vi "Dashboard Main.vi"() -> ()   [LabVIEW 2011]
uses:
  gun/gun_motor_state.ctl
  gun/gun_tracking_mode.ctl
  dashboard_data_gun_fast.ctl
  gun/gun_rt_slow_upstream_data.ctl
  idg_trust_t.ctl
  dashboard_data_drivetrain.ctl
  drivetrain/gear_shift_state.ctl
  drivetrain/gear_internal_shift_state.ctl
  roller/roller_internal_state.ctl
  roller/roller_user_state.ctl
  joe_johnson/joe_johnson_state.ctl
  2012vision/Vision Instrumentation Control.ctl
  dashboard_return_data.ctl
  2012vision/Camera State.ctl
  dashboard_globals.vi
  <vilib>/vision/NI_Vision_Development_Module.lvlib
panel:
  in  "open_logger":bool
  out "Automode":string
  out "gun tracking mode":T1
  out "Shooter Control Mode":T2
  out "Gun Power":dbl
  out "Gun Speed":dbl
  out "Gun Speed Target":dbl
  in  "Debug Mode":enum16{"Show Targets", "Show Lines", "Show All"}(ring)
  in  "Threshold Range":cluster{"Lower value":sgl, "Upper value":sgl}={"Lower value"=217.0, "Upper value"=255.0} {"Upper value" format="%.2f"; "Lower value" format="%.2f"}
  out "error out":errorcluster
  out "Image":T3(plugin-control)
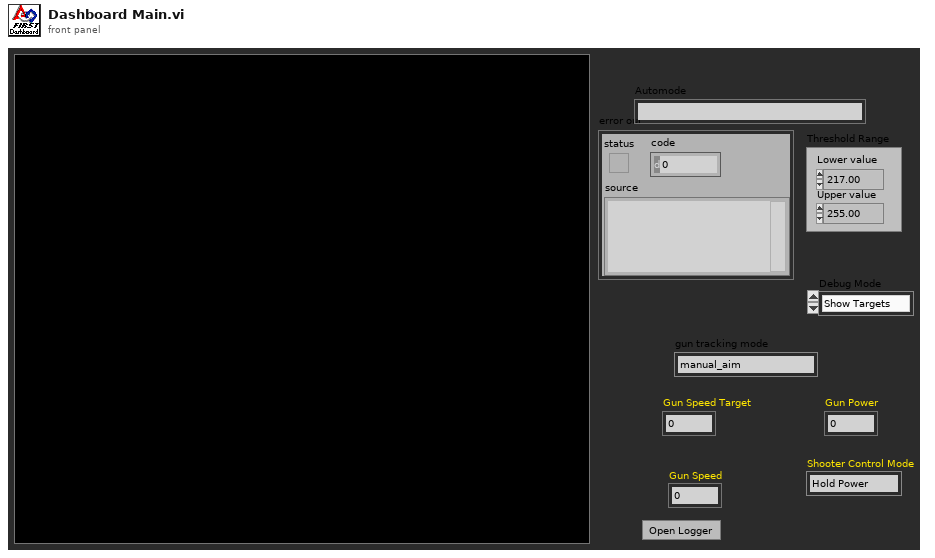
[diagram p1: front panel]
types:
  T1 = typedef "gun_tracking_mode.ctl" = enum16{"manual_aim", "auto_aim_camera", "preset_center_field", "preset_right_pocket", "preset_left_pocket", "align_center", "align_center_backwards", "auto_aim_key", "align_fold", "auton_custom", "preset_pass", "auto_aim_auton"}
  T2 = typedef "gun_motor_state.ctl" = enum16{"Hold Power", "Hold Speed", "Hold Distance", "Stop"}
  T3 = typedef "IMAQ Image.ctl" = refnum<image>
  T4 = typedef "dashboard_data_gun_fast.ctl" = cluster{"speed_setpoint":dbl, "speed_sensor":dbl, "gun_power":dbl, "gun_control_mode":T2, "gun_tracking_mode":T1}
  T5 = typedef "gun_rt_slow_upstream_data.ctl" = cluster{"turret":cluster{"turret_analog":dbl, "turret_angle":dbl, "turret_motor":dbl, "turret_idg_state":T6}, "hood":cluster{"hood_analog":dbl, "hood_angle":dbl, "hood_motor":dbl, "hood_idg_state":T6}}
  T6 = typedef "idg_trust_t.ctl" = enum16{"fault_move", "fault_high", "fault_low", "out_high", "out_low", "trust"}
  T7 = typedef "dashboard_data_drivetrain.ctl" = cluster{"left":cluster{"request":dbl, "enc_speed":dbl}, "right":cluster{"request":dbl, "enc_speed":dbl}, "gear shift state":T8, "gear shift internal state":T9}
  T8 = typedef "gear_shift_state.ctl" = enum16{"low", "high"}
  T9 = typedef "gear_internal_shift_state.ctl" = enum16{"low", "high", "low_peak", "high_peak"}
  T10 = typedef "roller_internal_state.ctl" = enum16{"idle", "bump", "full", "fire_intermediate", "fire_finish", "fire_entry", "fire_end", "fire_recover"}
  T11 = typedef "roller_user_state.ctl" = enum16{"off", "collect", "blow", "force suck"}
  T12 = typedef "joe_johnson_state.ctl" = enum16{"fold", "down", "up", "ramp", "bridge_lift", "manual", "ramp_stay"}
  T13 = cluster{"gun_fast":T4, "gun_slow":T5, "drivetrain_data":T7, "roller data":cluster{"roller internal state":T10, "roller user state":T11, "sws":cluster{"r_sw_b1":bool, "r_sw_b2":bool, "r_sw_b3":bool, "r_sw_gun":bool, "r_sw_low":bool}}, "joe_johnson_data":cluster{"analog":dbl, "input":dbl, "joe_johnson_state":T12, "idg_state":T6}}
  T14 = typedef "Image Type" = u32
  T15 = typedef "LVRectTypeDef.ctl" = cluster{"left":i16, "top":i16, "right":i16, "bottom":i16}
  T16 = cluster{"Competition mode":bool, "Robot Link":bool, "Autonomous":bool, "Enabled":bool, "E-Stop":bool}
  T17 = typedef "Vision Instrumentation Control.ctl" = cluster{"Draw Boxes":bool, "Draw Scores":bool, "Draw Lines":bool, "Draw Line Angles":bool, "Draw Targets":bool, "Draw Compound Crosshair":bool, "Draw Center Line":bool}
  T18 = enum32{"AutoM", "Close", "Dilate", "Erode", "Gradient", "Gradient in", "Gradient out", "HitMiss", "Open", "PClose", "POpen", "Thick", "Thin"}
  T19 = typedef "dashboard_return_data.ctl" = cluster{"Targetting Output":cluster{"X Position":dbl, "Distance":dbl, "Camera State":T20}, "Camera Error Status":errorcluster, "packet send timestamp":u32, "img process timestamp":u32}
  T20 = typedef "Camera State.ctl" = enum16{"No Targets", "Low Confidence", "Medium Confidence", "High Confidence", "Camera Error"}
  T21 = cluster{"Rect Coverage":dbl, "Aspect Ratio":dbl, "X Edge Strength":dbl, "Y Edge Strength":dbl}
  T22 = typedef "WPI_CameraImageSize.ctl" = enum16{"640x480", "320x240", "160x120"}
  T23 = cluster{"fps dashboard":i32, "compression dashboard":i32, "img size dashboard":T22}
  T24 = cluster{cluster{"Left":dbl, "Top":dbl, "Right":dbl, "Bottom":dbl}, cluster{"Score":dbl, "Score":dbl, "X Score":dbl, "Y Score":dbl}, "Clipped Edge":cluster{"Left":bool, "Top":bool, "Right":bool, "Bottom":bool}}[]
  T25 = cluster{"X Position":dbl, "Distance":dbl, "Camera State":T20}
  T26 = typedef "Diamond Target Output.ctl" = cluster{"Position":cluster{"X":dbl, "Y":dbl, "Distance":dbl}, "Est. Position":T27, "Target Confidence":T28}
  T27 = typedef "Rectangle Position.ctl" = enum16{"Unknown", "Top", "Right", "Left", "Bottom"}
  T28 = typedef "Target Confidence.ctl" = enum16{"Good", "Good-Clipped Y", "Marginal-Clipped X"}
  T29 = typedef "Line.ctl" = cluster{"First Point":cluster{"X":dbl, "Y":dbl, "Index":dbl}, "Second Point":cluster{"X":dbl, "Y":dbl, "Index":dbl}, "theta":dbl, "Direction":T30, "Line Confidence":T31}
  T30 = typedef "Direction.ctl" = enum16{"Rt", "Rt-Up", "Up", "Lt-Up", "Lt", "Lt-Dn", "Dn", "Rt-Dn", "Unknown"}
  T31 = typedef "Line Confidence.ctl" = enum16{"Good", "Bad"}
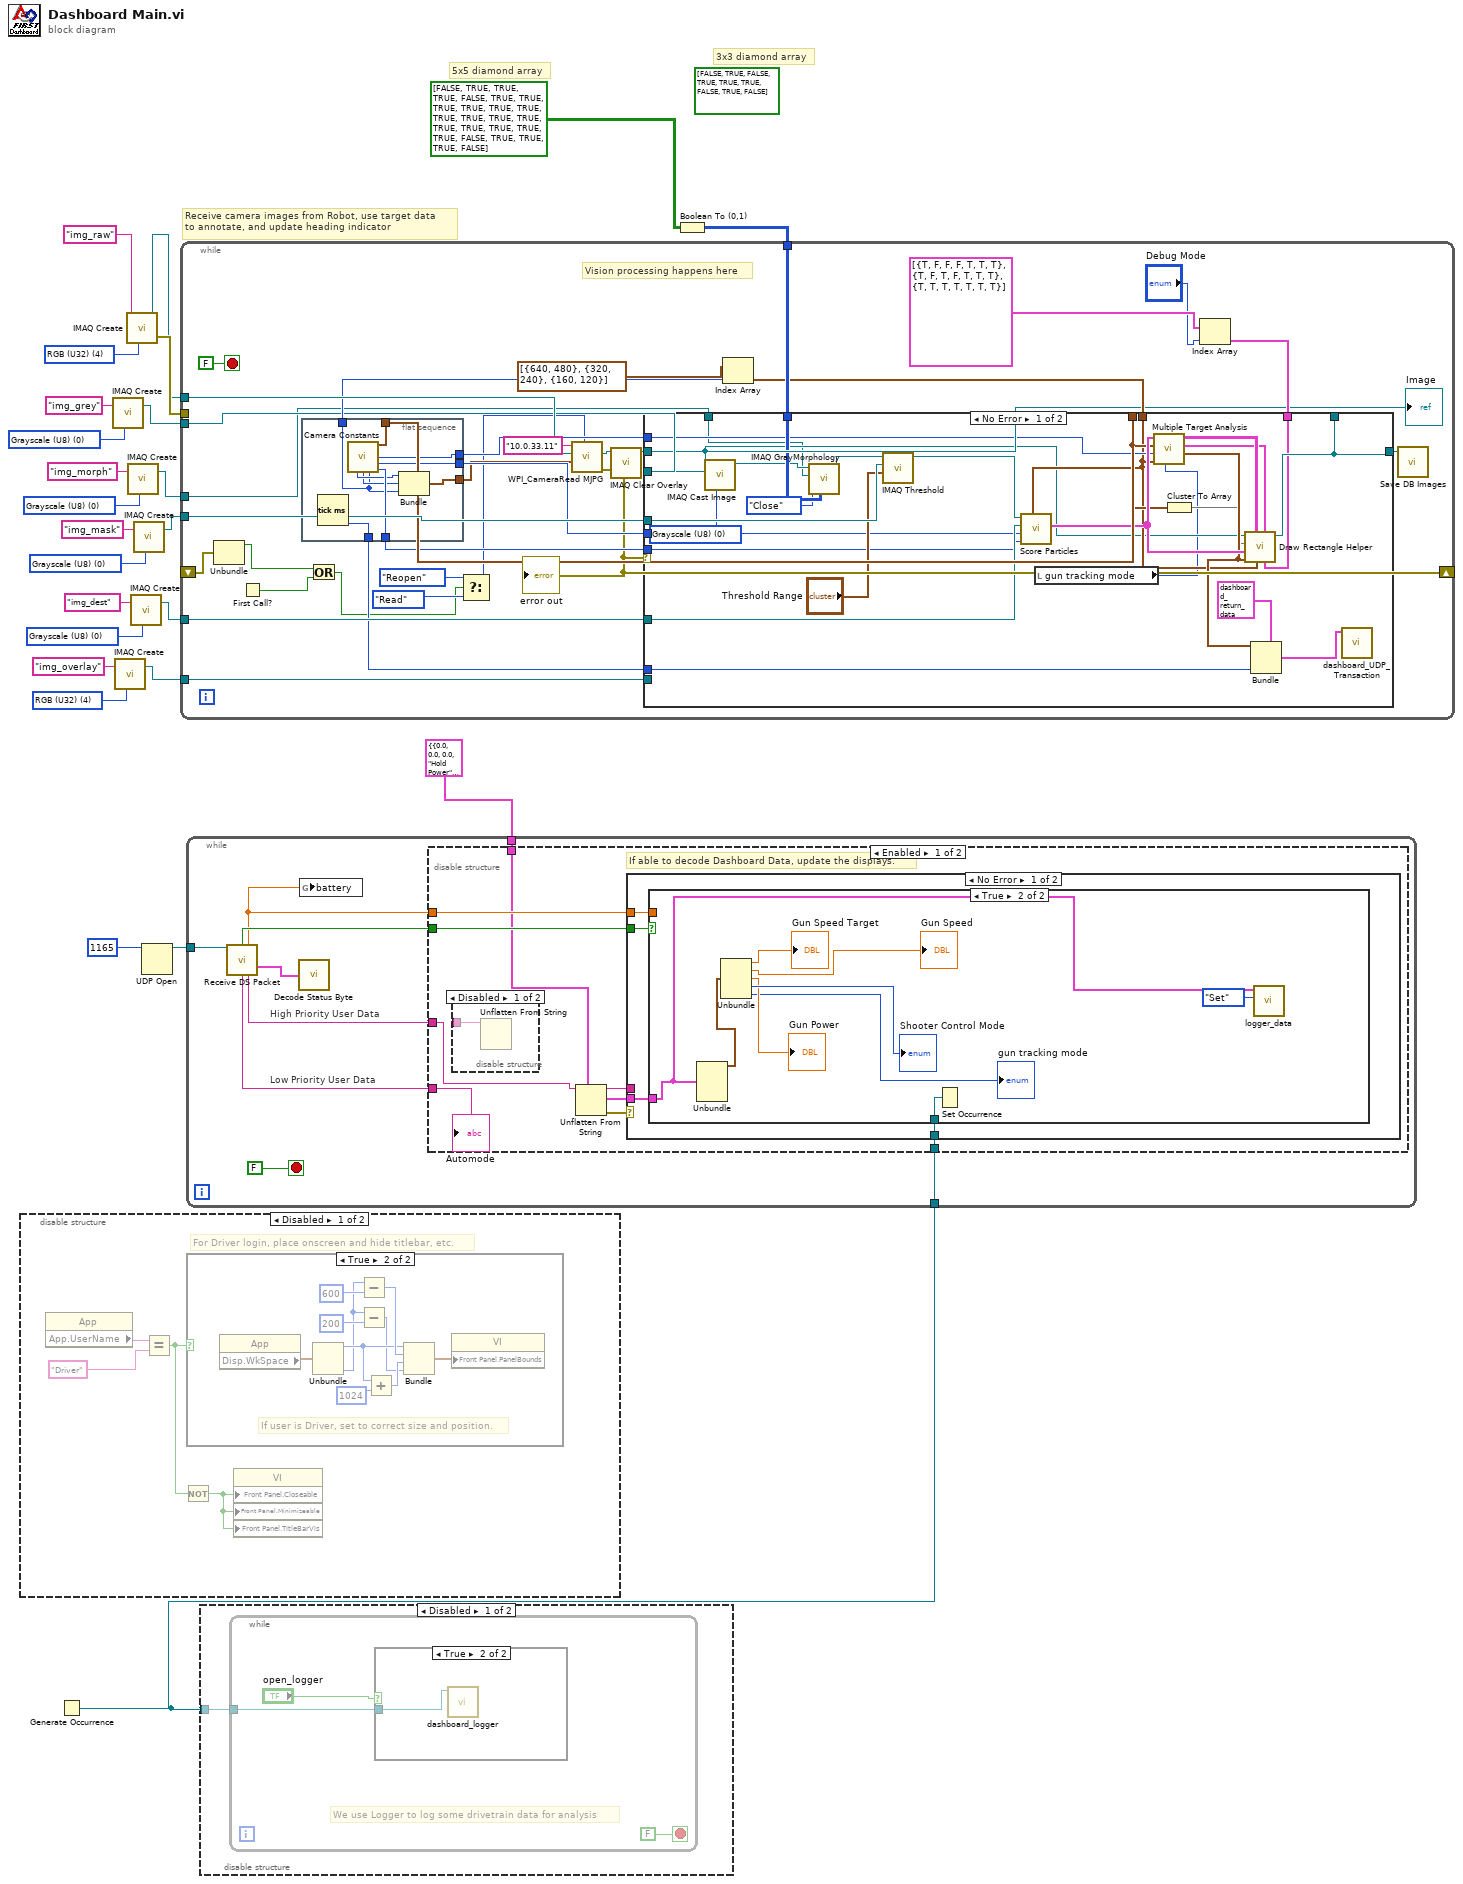
[diagram p0: block diagram]
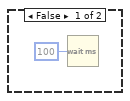
[diagram p2: hidden frame]
diagram:
  (unwired) bool[][] [[FALSE, TRUE, FALSE], [TRUE, TRUE, TRUE], [FALSE, TRUE, FALSE]]
  w5 = T14 4 items=["Grayscale (U8)", "Grayscale (I16)", "Grayscale (SGL)", "Complex (CSG)", "RGB (U32)", "HSL (U32)", "RGB (U64)"] ("Image Type")
  w8 = T14 0 items=["Grayscale (U8)", "Grayscale (I16)", "Grayscale (SGL)", "Complex (CSG)", "RGB (U32)", "HSL (U32)", "RGB (U64)"] ("Image Type")
  w12 = T14 0 items=["Grayscale (U8)", "Grayscale (I16)", "Grayscale (SGL)", "Complex (CSG)", "RGB (U32)", "HSL (U32)", "RGB (U64)"] ("Image Type")
  w22 = T14 0 items=["Grayscale (U8)", "Grayscale (I16)", "Grayscale (SGL)", "Complex (CSG)", "RGB (U32)", "HSL (U32)", "RGB (U64)"] ("Image Type")
  w19 = T14 0 items=["Grayscale (U8)", "Grayscale (I16)", "Grayscale (SGL)", "Complex (CSG)", "RGB (U32)", "HSL (U32)", "RGB (U64)"] ("Image Type")
  w15 = T14 4 items=["Grayscale (U8)", "Grayscale (I16)", "Grayscale (SGL)", "Complex (CSG)", "RGB (U32)", "HSL (U32)", "RGB (U64)"] ("Image Type")
  # "3x3 diamond array"
  # "5x5 diamond array"
  # "Receive camera images from Robot, use target data\nto annotate, and update heading indicator"
  n1 = disable-structure shown="Disabled" {
    frame Disabled {
      # "For Driver login, place onscreen and hide titlebar, etc."
      n2 = property class="App"() -> ("App.UserName"=w28:string)  [unwired: 2 in, 2 out]
      n3 = Equal?(x=w28, y="Driver") -> (x = y?=w27:bool)
      n4 = Not(x=w27) -> (.not. x?=w26:bool)
      n5 = case shown="True" w27 {
        frame False {
        }
        frame True {
          # "If user is Driver, set to correct size and position."
          n6 = property class="App"() -> ("Disp.WkSpace"=w39:T15)  [unwired: 2 in, 2 out]
          n7 = Unbundle(w39) -> ("left"=w34:i16, "bottom"=w30:i16)  [unwired: 2 out]
          n8 = Subtract(x=w30, y=600) -> (x-y=w36:i32)
          n9 = Subtract(x=w30, y=200) -> (x-y=w31:i32)
          n10 = Add(x=w34, y=1024) -> (x+y=w35:i32)
          n11 = Bundle("left"=w34, w36, w35, w31) -> (w38:cluster{"left":i16, i32, i32, i32})  [unwired: 1 out]
          n12 = property class="VI"("Front Panel.PanelBounds"=w38) -> ()  [unwired: 2 in, 2 out]
        }
      }
      n13 = property class="VI"("Front Panel.Closeable"=w26, "Front Panel.Minimizeable"=w26, "Front Panel.TitleBarVis"=w26) -> ()  [unwired: 2 in, 2 out]
    }
    frame Enabled {
    }
  }
  n14 = Generate Occurrence() -> (w1:refnum<k4>)
  n15 = call "IMAQ Create"("Image Name"="img_grey", "Image Type"=w8) -> ("New Image"=w7:T3)  [unwired: 2 in, 2 out]
  n16 = call "IMAQ Create"("Image Name"="img_overlay", "Image Type"=w5) -> ("New Image"=w4:T3)  [unwired: 2 in, 2 out]
  n17 = call "IMAQ Create"("Image Name"="img_raw", "Image Type"=w15) -> ("New Image"=w17:T3, "error out"=w18:errorcluster)  [unwired: 2 in, 1 out]
  n18 = call "IMAQ Create"("Image Name"="img_morph", "Image Type"=w19) -> ("New Image"=w21:T3)  [unwired: 2 in, 2 out]
  n19 = call "IMAQ Create"("Image Name"="img_dest", "Image Type"=w12) -> ("New Image"=w11:T3)  [unwired: 2 in, 2 out]
  n20 = call "IMAQ Create"("Image Name"="img_mask", "Image Type"=w22) -> ("New Image"=w14:T3)  [unwired: 2 in, 2 out]
  n21 = UDP Open(11:u16 1165 ("port")) -> (port=w24:refnum<k16>)  [unwired: 2 in, 4 out]
  n22 = while {
    tunnel: w24 -> [w46]
    tunnel: T13 {"gun_fast"={"speed_setpoint"=0.0, "speed_sensor"=0.0, "gun_power"=0.0, "gun_control_mode"=enum."Hold Power", "gun_tracking_mode"=enum."manual_aim"}, "gun_slow"={"turret"={"turret_analog"=0.0, "turret_angle"=0.0, "turret_motor"=0.0, "turret_idg_state"=enum."fault_high"}, "hood"={"hood_analog"=0.0, "hood_angle"=0.0, "hood_motor"=0.0, "hood_idg_state"=enum."fault_high"}}, "drivetrain_data"={"left"={"request"=0.0, "enc_speed"=0.0}, "right"={"request"=0.0, "enc_speed"=0.0}, "gear shift state"=enum."low", "gear shift internal state"=enum."low"}, "roller data"={"roller internal state"=enum."idle", "roller user state"=enum."off", "sws"={"r_sw_b1"=FALSE, "r_sw_b2"=FALSE, "r_sw_b3"=FALSE, "r_sw_gun"=FALSE, "r_sw_low"=FALSE}}, "joe_johnson_data"={"analog"=0.0, "input"=0.0, "joe_johnson_state"=enum."fold", "idg_state"=enum."fault_high"}} ("Cluster") -> [w42]
    tunnel: w1 -> [w41]
    stop <- FALSE stop-if-true
    # "High Priority User Data"
    # "Low Priority User Data"
    n23 = call "Receive DS Packet.vi"("Recv Socket"=w46) -> ("New Dashboard Data"=w45:bool, "Battery"=w40:sgl, "Status"=w47:T16, "Low Priority User Data"=w44:string, "High Priority User Data"=w43:string)  [unwired: 1 in, 9 out]
    n24 = call "Decode Status Byte.vi"("Status Byte"=w47) -> ()  [unwired: 2 out]
    n25 = global write "dashboard_globals.vi" "battery"(w40) -> ()
    n26 = disable-structure shown="Enabled" {
      disable-tunnel: w45 -> [w55 _]
      disable-tunnel: w44 -> [w50 _]
      disable-tunnel: w43 -> [w52 _]
      disable-tunnel: w40 -> [w53 _]
      disable-tunnel: w42 -> [w51 _]
      disable-tunnel: w41 -> [w49 _]
      frame Enabled {
        # "If able to decode Dashboard Data, update the displays."
        n27 = disable-structure shown="Disabled" {
          disable-tunnel: _ -> [w58 _]
          frame Disabled {
            n28 = Unflatten From String(binary string=w58) -> ()  [unwired: 2 in, 5 out]
          }
          frame Enabled {
          }
        }
        n29 = Unflatten From String(type=w51, binary string=w52) -> (rest of the binary string=w54:string, value=w57:T13, error out=w56:errorcluster)  [unwired: 1 in, 2 out]
        n30 = case shown="No Error" w56 {
          tunnel: w57 -> [w62 _]
          tunnel: w55 -> [w61 _]
          tunnel: w54 -> [_ _]
          tunnel: w53 -> [w60 _]
          tunnel: w49 -> [w59 _]
          frame No Error {
            n31 = case shown="True" w61 {
              tunnel: w62 -> [_ w64]
              tunnel: w60 -> [_ _]
              tunnel: w59 -> [_ w66]
              frame False {
                # "Don't update if the robot hasn't sent new data"
              }
              frame True {
                n32 = Unbundle(w64) -> ("gun_fast"=w65:T4)  [unwired: 4 out]
                n33 = Unbundle(w65) -> ("speed_setpoint"=→"Gun Speed Target":dbl, "speed_sensor"=→"Gun Speed":dbl, "gun_power"=→"Gun Power":dbl, "gun_control_mode"=→"Shooter Control Mode":T2, "gun_tracking_mode"=→"gun tracking mode":T1)
                n34 = Set Occurrence(w66) -> ()
                n35 = call "logger_data.vi"("data_store_mode"=enum16{"Set", "Get"}."Set", "dashboard_data"=w64) -> ()  [unwired: 9 in, 1 out]
              }
            }
          }
          frame Error {
            # "Your datatypes don't match. The Dashboard Datatype.ctl in your Robot project\nand the big constant to the left of the loop need to match."
          }
        }
        "Automode" <- w50
      }
      frame Disabled {
      }
    }
  }
  n36 = disable-structure shown="Disabled" {
    disable-tunnel: w1 -> [w72 _]
    frame Disabled {
      n37 = while {
        tunnel: w72 -> [w73]
        stop <- FALSE stop-if-true
        # "We use Logger to log some drivetrain data for analysis"
        n38 = case shown="True" "open_logger" {
          tunnel: w73 -> [_ w77]
          frame False {
            n39 = Wait (ms)(milliseconds to wait=u32 100) -> ()  [unwired: 1 out]
          }
          frame True {
            n40 = call "dashboard_logger.vi"("data occurrence"=w77) -> ()  [unwired: 11 in]
          }
        }
      }
    }
    frame Enabled {
    }
  }
  n41 = Boolean To (0,1)(Boolean=bool[][] [[FALSE, TRUE, TRUE, TRUE, FALSE], [TRUE, TRUE, TRUE, TRUE, TRUE], [TRUE, TRUE, TRUE, TRUE, TRUE], [TRUE, TRUE, TRUE, TRUE, TRUE], [FALSE, TRUE, TRUE, TRUE, FALSE]]) -> (0, 1=w10:i16[][])
  n42 = while {
    tunnel: w17 -> [w108]
    tunnel: w18 -> [_]
    tunnel: w21 -> [w91]
    tunnel: w10 -> [w101]
    tunnel: w14 -> [w105]
    tunnel: w11 -> [w104]
    tunnel: w7 -> [w92]
    tunnel: w4 -> [w87]
    shift-right: [w86] -> _
    shift-left: _ -> [w85]
    stop <- FALSE stop-if-true
    # "Vision processing happens here"
    n43 = Unbundle(w85) -> ("status"=w83:bool)  [unwired: 2 out]
    n44 = First Call?() -> (First Call?: T/F=w84:bool)
    n45 = flat-sequence {
      tunnel: [w147] -> w102
      tunnel: [w146] -> w100
      tunnel: [w145] -> w99
      tunnel: [w144] -> w98
      tunnel: [w143] -> w97
      tunnel: [w140] -> w96
      tunnel: [w139] -> w94
      frame #0 {
        n46 = Tick Count (ms)() -> (millisecond timer value=w147:u32)
        n47 = call "Camera Constants.vi"() -> ("score limits"=w146:T21, "cam type"=w140:enum16{"206", "1011"}, "particle count limit"=w145:i32, "fps dashboard"=w142:i32, "compression dashboard"=w141:i32, "img size dashboard"=w139:T22, "area size limit"=w144:i32)  [unwired: 5 in, 4 out]
        n48 = Bundle("fps dashboard"=w142, "compression dashboard"=w141, "img size dashboard"=w139) -> (w143:T23)  [unwired: 1 in]
      }
    }
    n49 = Or(x=w83, y=w84) -> (x .or. y?=w82:bool)
    n50 = Select(t=enum16{"Read", "Reopen", "Close"}."Reopen", s=w82, f=enum16{"Read", "Reopen", "Close"}."Read" ("Operation")) -> (s? t:f=w89:enum16{"Read", "Reopen", "Close"})
    n51 = call <vilib>:"WPI_CameraRead MJPG.vi"("Operation"=w89, "Camera Settings"=w97, "Image"=w108, "address"="10.0.33.11") -> ("error out"=w86:errorcluster, "Image Out"=w107:T3)  [unwired: 6 in]
    "error out" <- w86
    n52 = call "IMAQ Clear Overlay"("Image"=w107) -> ("Image Out"=w78:T3)  [unwired: 2 in, 8 out]
    "Image" <- w78
    n53 = Index Array(array=cluster{i32, i32}[] [{640, 480}, {320, 240}, {160, 120}], index=w94) -> (element=w93:cluster{i32, i32})
    n54 = Index Array(array=T17[] [{"Draw Boxes"=TRUE, "Draw Scores"=FALSE, "Draw Lines"=FALSE, "Draw Line Angles"=FALSE, "Draw Targets"=TRUE, "Draw Compound Crosshair"=TRUE, "Draw Center Line"=TRUE}, {"Draw Boxes"=TRUE, "Draw Scores"=FALSE, "Draw Lines"=TRUE, "Draw Line Angles"=FALSE, "Draw Targets"=TRUE, "Draw Compound Crosshair"=TRUE, "Draw Center Line"=TRUE}, {"Draw Boxes"=TRUE, "Draw Scores"=TRUE, "Draw Lines"=TRUE, "Draw Line Angles"=TRUE, "Draw Targets"=TRUE, "Draw Compound Crosshair"=TRUE, "Draw Center Line"=TRUE}], index="Debug Mode") -> (element=w79:T17)
    n55 = case shown="No Error" w86 {
      tunnel: w105 -> [w136 _]
      tunnel: w104 -> [w133 _]
      tunnel: [w113 w138] -> w103
      tunnel: w102 -> [w126 _]
      tunnel: w101 -> [w125 _]
      tunnel: w100 -> [w123 _]
      tunnel: w99 -> [w122 _]
      tunnel: w98 -> [w121 _]
      tunnel: w96 -> [w120 _]
      tunnel: w93 -> [w119 _]
      tunnel: [w113 w138] -> _
      tunnel: w78 -> [w118 _]
      tunnel: w92 -> [w115 _]
      tunnel: w91 -> [w114 w138]
      tunnel: w87 -> [_ _]
      tunnel: w79 -> [w112 _]
      frame No Error {
        w116 = T14 0 items=["Grayscale (U8)", "Grayscale (I16)", "Grayscale (SGL)", "Complex (CSG)", "RGB (U32)", "HSL (U32)", "RGB (U64)", "Grayscale (U16)"] ("Image Type")
        n56 = call "IMAQ Cast Image"("Image Type"=w116, "Image Dst"=w115, "Image Src"=w118) -> ("Image Dst Out"=w117:T3)  [unwired: 7 in, 1 out]
        n57 = call "IMAQ GrayMorphology"("Structuring Element"=w125, "Operation"=T18."Close", "Image Dst"=w114, "Image Src"=w117) -> ("Image Dst Out"=w137:T3)  [unwired: 6 in, 1 out]
        n58 = call "IMAQ Threshold"("Range"="Threshold Range", "Image Dst"=w136, "Image Src"=w137) -> ("Image Dst Out"=w134:T3)  [unwired: 7 in, 1 out]
        n59 = call "Score Particles.vi"("Image Size"=w119, "Area Size Limit"=w121, "Particle Count Limit"=w122, "Image Dst"=w133, "Image Refnum in"=w134) -> ("Targets"=w130:T24)  [unwired: 5 in, 1 out]
        n60 = local read "gun tracking mode"() -> (w111:T1)
        n61 = call "Multiple Target Analysis.vi"("gun tracking mode"=w111, "Image Size"=w119, "Camera Type"=w120, "Score Limits"=w123, "Targets"=w130) -> ("Targetting Output"=w127:T25, "Diamond Targets"=w131:T26[], "Lines"=w132:T29[][])  [unwired: 4 in]
        n62 = Cluster To Array(cluster=w123) -> (array=w124:dbl[])
        n63 = call "Draw Rectangle Helper.vi"("Vision Instrumentation"=w112, "Diamond Targets"=w131, "Image Size"=w119, "Lines"=w132, "Targetting Output"=w127, "Targets"=w130, "Score Limits"=w124, "Refnum in"=w118) -> ("Refnum out"=w113:T3)  [unwired: 3 in]
        n64 = Bundle(cluster=T19 {"Targetting Output"={"X Position"=0.0, "Distance"=0.0, "Camera State"=enum."No Targets"}, "Camera Error Status"={"status"=FALSE, "code"=0, "source"=""}, "packet send timestamp"=0, "img process timestamp"=0} ("Dashboard Return Data"), "Targetting Output"=w127, "img process timestamp"=w126) -> (w128:T19)  [unwired: 2 in]
        n65 = call "dashboard_UDP_Transaction.vi"("Dashboard Return Data"=w128) -> ()  [unwired: 11 in]
      }
      frame Error {
      }
    }
    n66 = call "Save DB Images.vi"("Image"=w103) -> ()  [unwired: 2 in, 1 out]
  }
